vi "Heila IQ Optimization.vi"(4 "Invert":bool, 6 "Index":bool, 8 "error in (no error)":errorcluster, 9 "Dispatch":bool, 10 "Price":sgl[](array[numeric]), 11 "Modbus master in":refnum<class "Modbus Master.lvclass">) -> (0 "error out":errorcluster, 2 "Output Variables":sgl[](array[numeric]), 3 "Modbus master out":refnum<class "Modbus Master.lvclass">)   [LabVIEW 2019]
uses:
  <vilib>/Modbus/master/Modbus Master.lvclass
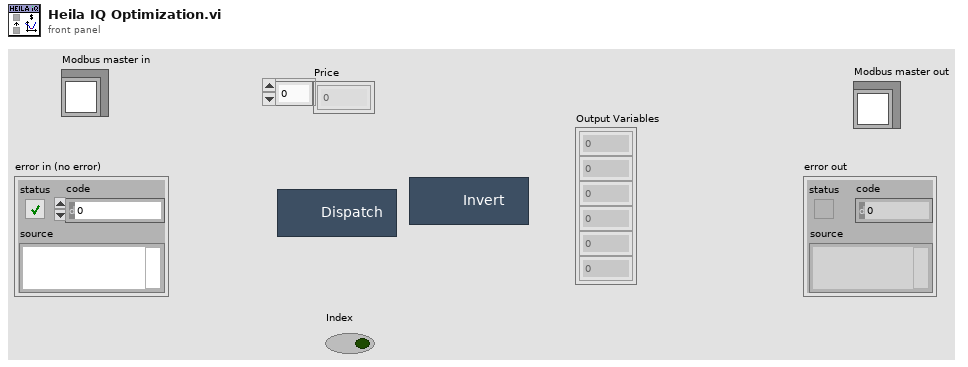
[diagram p1: front panel]
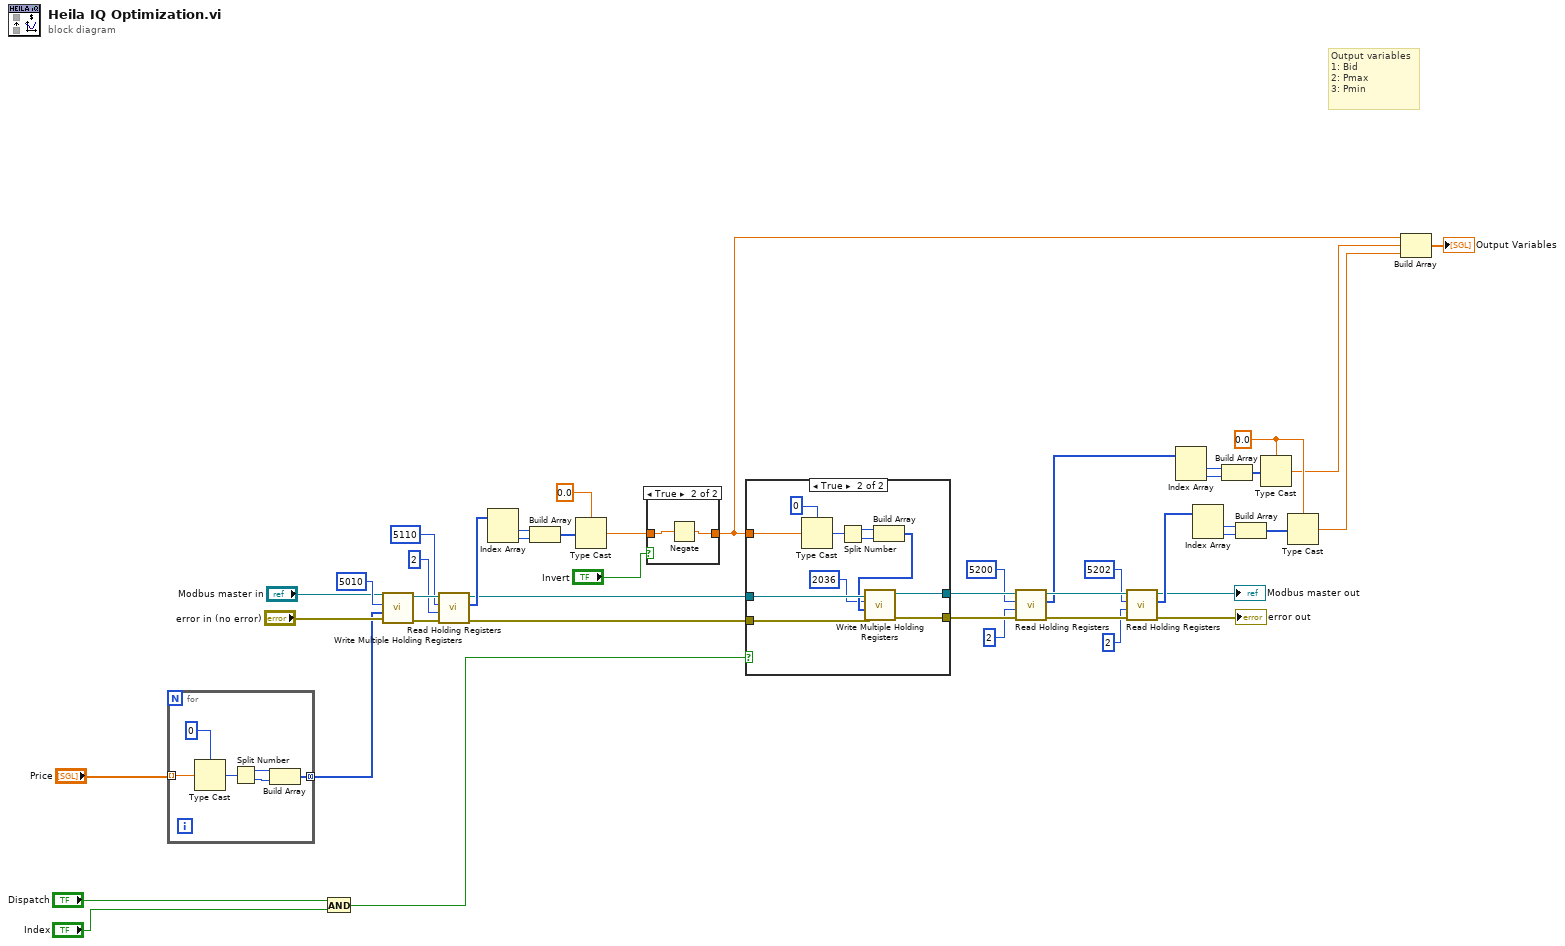
[diagram p0: block diagram]
diagram:
  w14 = sgl 0.0
  # "Output variables\n1: Bid\n2: Pmax\n3: Pmin"
  n1 = for {
    tunnel: [w46] -> w7 mode=concatenating
    tunnel: "Price" -> [w45] mode=indexing
    n2 = Type Cast(type=u32 0, x=w45) -> (*(type *) &x=w50:u32)
    n3 = Split Number(x=w50) -> (hi(x)=w48:u16, lo(x)=w47:u16)
    n4 = Build Array(w48, w47) -> (w46:u16[])
  }
  n5 = And(x="Dispatch", y="Index") -> (x .and. y?=w4:bool)
  n6 = call-dynamic "Write Multiple Holding Registers.vi"("error in (no error)"="error in (no error)", "holding register values"=w7, "starting address"=u16 5010, "Modbus master in"="Modbus master in") -> ("error out"=w42:errorcluster, "Modbus master out"=w43:refnum<class "Modbus Master.lvclass">)  [unwired: 6 in]
  n7 = call-dynamic "Read Holding Registers.vi"("error in (no error)"=w42, "number of holding registers"=u16 2, "starting address"=u16 5110, "Modbus master in"=w43) -> ("error out"=w33:errorcluster, "register values"=w39:u16[], "Modbus master out"=w34:refnum<class "Modbus Master.lvclass">)  [unwired: 5 in]
  n8 = Index Array(array=w39) -> (element #1=w38:u16, element #2=w37:u16)  [unwired: 2 in]
  n9 = Build Array(w38, w37) -> (w36:u16[])
  n10 = Type Cast(type=sgl 0.0, x=w36) -> (*(type *) &x=w3:sgl)
  n11 = case shown="True" "Invert" {
    tunnel: w3 -> [w51 w53]
    tunnel: [w51 w52] -> w1
    frame False {
    }
    frame True {
      n12 = Negate(x=w53) -> (-x=w52:sgl)
    }
  }
  n13 = case shown="True" w4 {
    tunnel: w34 -> [w55 w66]
    tunnel: w33 -> [w54 w59]
    tunnel: w1 -> [_ w61]
    tunnel: [w55 w57] -> w32
    tunnel: [w54 w56] -> w31
    frame False {
    }
    frame True {
      n14 = Type Cast(type=u32 0, x=w61) -> (*(type *) &x=w65:u32)
      n15 = Split Number(x=w65) -> (hi(x)=w63:u16, lo(x)=w62:u16)
      n16 = Build Array(w63, w62) -> (w60:u16[])
      n17 = call-dynamic "Write Multiple Holding Registers.vi"("error in (no error)"=w59, "holding register values"=w60, "starting address"=u16 2036, "Modbus master in"=w66) -> ("error out"=w56:errorcluster, "Modbus master out"=w57:refnum<class "Modbus Master.lvclass">)  [unwired: 6 in]
    }
  }
  n18 = call-dynamic "Read Holding Registers.vi"("error in (no error)"=w31, "number of holding registers"=u16 2, "starting address"=u16 5200, "Modbus master in"=w32) -> ("error out"=w28:errorcluster, "register values"=w21:u16[], "Modbus master out"=w27:refnum<class "Modbus Master.lvclass">)  [unwired: 5 in]
  n19 = call-dynamic "Read Holding Registers.vi"("error in (no error)"=w28, "number of holding registers"=u16 2, "starting address"=u16 5202, "Modbus master in"=w27) -> ("error out"=→"error out":errorcluster, "register values"=w17:u16[], "Modbus master out"=→"Modbus master out":refnum<class "Modbus Master.lvclass">)  [unwired: 5 in]
  n20 = Index Array(array=w21) -> (element #1=w24:u16, element #2=w23:u16)  [unwired: 2 in]
  n21 = Index Array(array=w17) -> (element #1=w20:u16, element #2=w19:u16)  [unwired: 2 in]
  n22 = Build Array(w24, w23) -> (w22:u16[])
  n23 = Build Array(w20, w19) -> (w18:u16[])
  n24 = Type Cast(type=w14, x=w22) -> (*(type *) &x=w13:sgl)
  n25 = Type Cast(type=w14, x=w18) -> (*(type *) &x=w12:sgl)
  n26 = Build Array(w1, w13, w12) -> (→"Output Variables":sgl[])
